vi "Encoder_Var.vi"(2 "Drive_En_Reset":bool, 3 "DIO":T1) -> (0 "Encoder_Var":T10)   [LabVIEW 2015]
uses:
  Ref_Num/DIO_Type_Def.ctl
  <vilib>/Rock Robotics/WPI/Ultrasonic/WPI_SonarMB1010DigitalDeviceRef.ctl
  <vilib>/Rock Robotics/WPI/Counter/WPI_CounterDevRef.ctl
  <vilib>/Rock Robotics/SystemInterfaces/Counter/FPGA_CounterCtrSystemIndex.ctl
  <vilib>/Rock Robotics/WPI/Encoder/WPI_EncoderDevRef.ctl
  <vilib>/Rock Robotics/SystemInterfaces/Encoder/FPGA_EncoderIdx.ctl
  <vilib>/Rock Robotics/WPI/Encoder/WPI_EncoderType.ctl
  <vilib>/Rock Robotics/WPI/DigitalInput/WPI_DigitalInputDevRef.ctl
  <vilib>/Rock Robotics/SystemInterfaces/DIO/FPGA_DIOChannel.ctl
  Global_Var/Drive_Global.vi
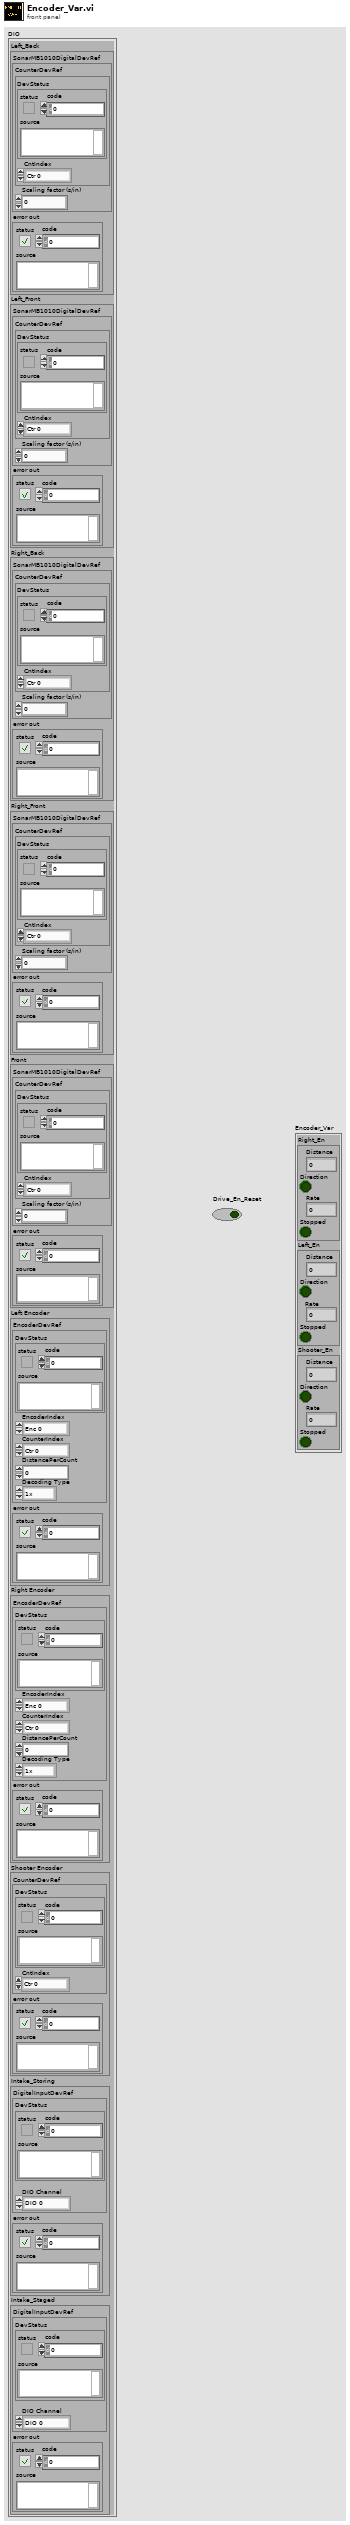
[diagram p1: front panel]
types:
  T1 = typedef "DIO_Type_Def.ctl" = cluster{"Left_Back":cluster{"SonarMB1010DigitalDevRef":T2, "error out":errorcluster}, "Left_Front":cluster{"SonarMB1010DigitalDevRef":T2, "error out":errorcluster}, "Right_Back":cluster{"SonarMB1010DigitalDevRef":T2, "error out":errorcluster}, "Right_Front":cluster{"SonarMB1010DigitalDevRef":T2, "error out":errorcluster}, "Front":cluster{"SonarMB1010DigitalDevRef":T2, "error out":errorcluster}, "Left Encoder":cluster{"EncoderDevRef":T5, "error out":errorcluster}, "Right Encoder":cluster{"EncoderDevRef":T5, "error out":errorcluster}, "Shooter Encoder":cluster{"CounterDevRef":T3, "error out":errorcluster}, "Intake_Storing":cluster{"DigitalInputDevRef":T8, "error out":errorcluster}, "Intake_Staged":cluster{"DigitalInputDevRef":T8, "error out":errorcluster}}
  T2 = typedef "WPI_SonarMB1010DigitalDeviceRef.ctl" = cluster{"CounterDevRef":T3, "Scaling factor (s/in)":dbl}
  T3 = typedef "WPI_CounterDevRef.ctl" = cluster{"DevStatus":errorcluster, "CntIndex":T4}
  T4 = typedef "FPGA_CounterCtrSystemIndex.ctl" = enum8{"Ctr 0", "Ctr 1", "Ctr 2", "Ctr 3", "Ctr 4", "Ctr 5", "Ctr 6", "Ctr 7", "Invalid"}
  T5 = typedef "WPI_EncoderDevRef.ctl" = cluster{"DevStatus":errorcluster, "EncoderIndex":T6, "CounterIndex":T4, "DistancePerCount":dbl, "Decoding Type":T7}
  T6 = typedef "FPGA_EncoderIdx.ctl" = enum8{"Enc 0", "Enc 1", "Enc 2", "Enc 3", "Enc 4", "Enc 5", "Enc 6", "Enc 7", "Invalid"}
  T7 = typedef "WPI_EncoderType.ctl" = enum16{"1x", "2x", "4x"}
  T8 = typedef "WPI_DigitalInputDevRef.ctl" = cluster{"DevStatus":errorcluster, "DIO Channel":T9}
  T9 = typedef "FPGA_DIOChannel.ctl" = enum8{"DIO 0", "DIO 1", "DIO 2", "DIO 3", "DIO 4", "DIO 5", "DIO 6", "DIO 7", "DIO 8", "DIO 9", "DIO MXP 0", "DIO MXP 1", "DIO MXP 2", "DIO MXP 3", "DIO MXP 4", "DIO MXP 5", "DIO MXP 6", "DIO MXP 7", "DIO MXP 8", "DIO MXP 9", "DIO MXP 10", "DIO MXP 11", "DIO MXP 12", "DIO MXP 13", "DIO MXP 14", "DIO MXP 15", "Invalid"}
  T10 = cluster{"Right_En":cluster{"Distance":dbl, "Direction":bool, "Rate":dbl, "Stopped":bool}, "Left_En":cluster{"Distance":dbl, "Direction":bool, "Rate":dbl, "Stopped":bool}, "Shooter_En":cluster{"Distance":dbl, "Direction":bool, "Rate":dbl, "Stopped":bool}}
  T11 = cluster{"Distance":dbl, "Direction":bool, "Rate":dbl, "Stopped":bool}
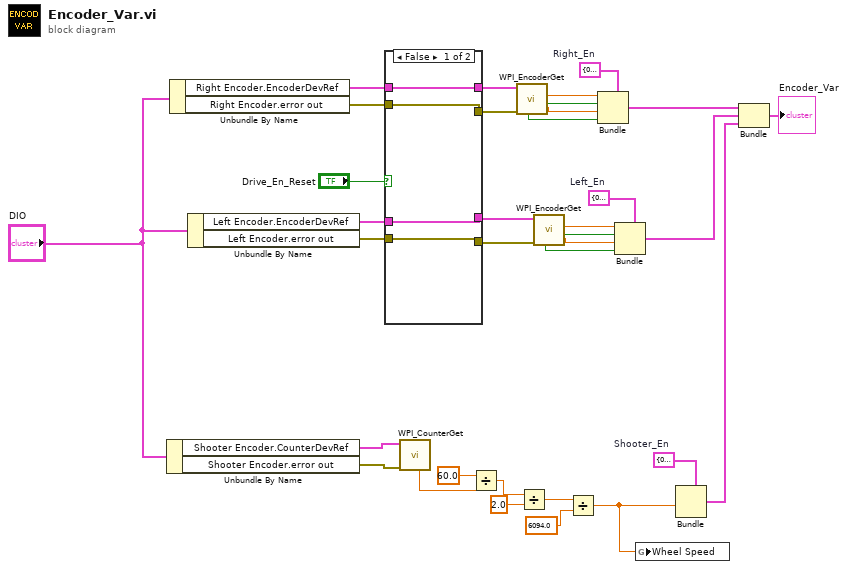
[diagram p0: block diagram]
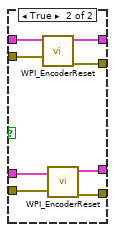
[diagram p2: hidden frame]
diagram:
  w15 = T11 {"Distance"=0.0, "Direction"=FALSE, "Rate"=0.0, "Stopped"=FALSE}  # Shooter_En
  w16 = T11 {"Distance"=0.0, "Direction"=FALSE, "Rate"=0.0, "Stopped"=FALSE}  # Left_En
  w17 = T11 {"Distance"=0.0, "Direction"=FALSE, "Rate"=0.0, "Stopped"=FALSE}  # Right_En
  n1 = Unbundle By Name("DIO") -> ("Shooter Encoder.CounterDevRef"=w9:T3, "Shooter Encoder.error out"=w8:errorcluster)
  n2 = Unbundle By Name("DIO") -> ("Right Encoder.EncoderDevRef"=w31:T5, "Right Encoder.error out"=w30:errorcluster)
  n3 = Unbundle By Name("DIO") -> ("Left Encoder.EncoderDevRef"=w29:T5, "Left Encoder.error out"=w28:errorcluster)
  n4 = case shown="False" "Drive_En_Reset" {
    tunnel: [w38 w46] -> w34
    tunnel: [w37 w45] -> w33
    tunnel: [w36 w44] -> w19
    tunnel: [w35 w43] -> w18
    tunnel: w31 -> [w38 w42]
    tunnel: w30 -> [w37 w41]
    tunnel: w29 -> [w36 w40]
    tunnel: w28 -> [w35 w39]
    frame False {
    }
    frame True {
      n5 = call <vilib>:"WPI_EncoderReset.vi"("error in (no error)"=w41, "EncoderDevRef"=w42) -> ("error out"=w45:errorcluster, "EncoderDevRef"=w46:T5)  [unwired: 8 in]
      n6 = call <vilib>:"WPI_EncoderReset.vi"("error in (no error)"=w39, "EncoderDevRef"=w40) -> ("error out"=w43:errorcluster, "EncoderDevRef"=w44:T5)  [unwired: 8 in]
    }
  }
  n7 = call <vilib>:"WPI_CounterGet.vi"("error in (no error)"=w8, "CounterDevRef in"=w9) -> ("Period (sec)"=w7:dbl)  [unwired: 4 in, 5 out]
  n8 = Divide(x=60.0, y=w7) -> (x/y=w5:dbl)
  n9 = call <vilib>:"WPI_EncoderGet.vi"("error in (no error)"=w33, "EncoderDevRef"=w34) -> ("Direction"=w26:bool, "Distance"=w27:dbl, "Rate"=w25:dbl, "Stopped"=w24:bool)  [unwired: 4 in, 2 out]
  n10 = Divide(x=w5, y=2.0) -> (x/y=w3:dbl)
  n11 = call <vilib>:"WPI_EncoderGet.vi"("error in (no error)"=w18, "EncoderDevRef"=w19) -> ("Direction"=w22:bool, "Distance"=w23:dbl, "Rate"=w21:dbl, "Stopped"=w20:bool)  [unwired: 4 in, 2 out]
  n12 = Divide(x=w3, y=6094.0) -> (x/y=w1:dbl)
  n13 = Bundle(cluster=w17, "Distance"=w27, "Direction"=w26, "Rate"=w25, "Stopped"=w24) -> (w14:T11)
  n14 = Bundle(cluster=w16, "Distance"=w23, "Direction"=w22, "Rate"=w21, "Stopped"=w20) -> (w13:T11)
  n15 = global write "Drive_Global.vi" "Wheel Speed"(w1) -> ()
  n16 = Bundle(cluster=w15, "Rate"=w1) -> (w12:T11)  [unwired: 3 in]
  n17 = Bundle("Right_En"=w14, "Left_En"=w13, "Shooter_En"=w12) -> (→"Encoder_Var":T10)  [unwired: 1 in]
